vi "ContinueCompare_DetectEvent.vi"(3 "status":bool, 4 "error in (no error)":errorcluster, 5 "Task ID":u32) -> (0 "continue compare data":T1, 1 "error out":errorcluster, 2 "Task ID out":u32)   [LabVIEW 2015]
panel:
  in  "pattern match count":i32
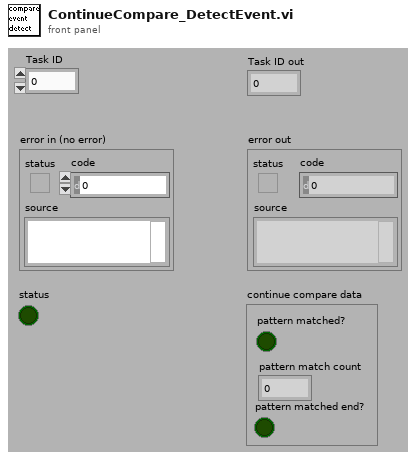
[diagram p1: front panel]
types:
  T1 = cluster{"pattern matched?":bool, "pattern matched end?":bool, "pattern match count":dbl}
  T2 = cluster{"pattern matched?":bool, "pattern matched end?":bool, "pattern match count":i32}
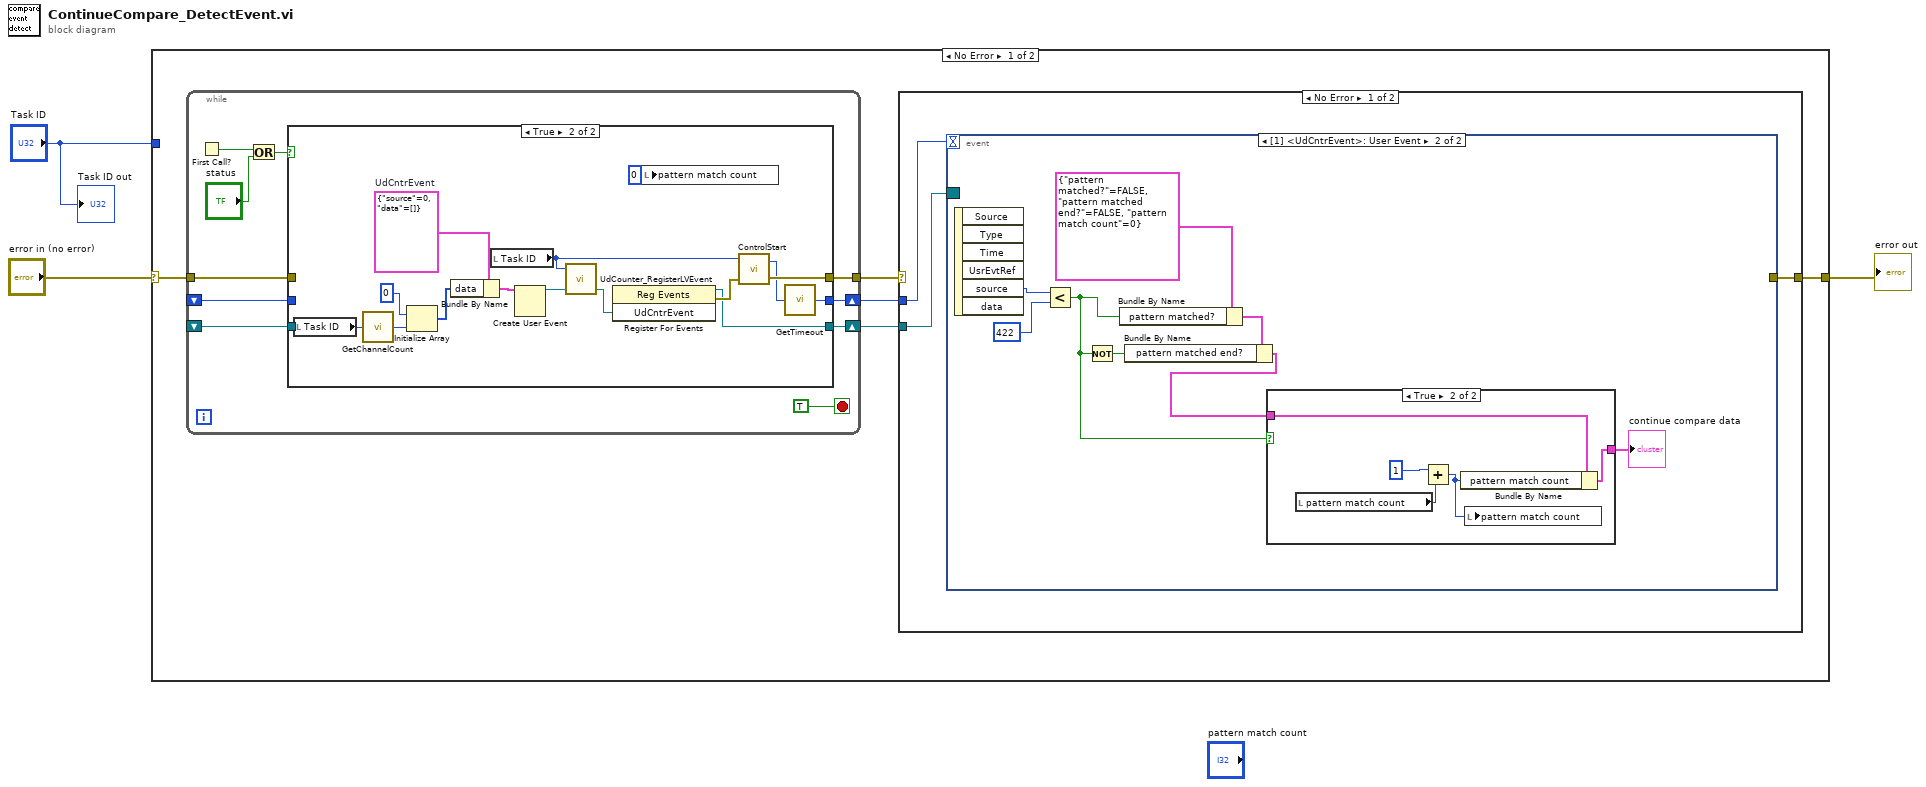
[diagram p0: block diagram]
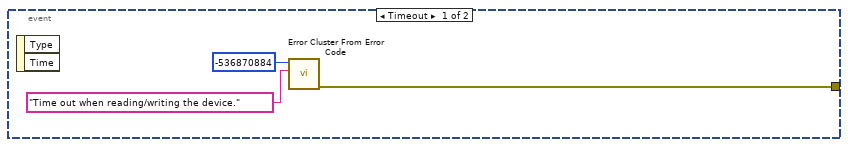
[diagram p2: hidden frame]
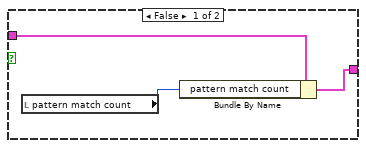
[diagram p3: hidden frame]
diagram:
  n1 = case shown="No Error" "error in (no error)" {
    selector: "error in (no error)" -> [w8 w60]
    tunnel: [w6 w60] -> w2
    tunnel: "Task ID" -> [_ _]
    frame No Error {
      n2 = while {
        tunnel: w8 -> [w37]
        tunnel: [w36] -> w7
        shift-right: [w34] -> w4
        shift-left: _ -> [w35]
        shift-right: [w32] -> w5
        shift-left: _ -> [w33]
        stop <- TRUE stop-if-true
        n3 = First Call?() -> (First Call?: T/F=w40:bool)
        n4 = Or(x=w40, y="status") -> (x .or. y?=w38:bool)
        n5 = case shown="True" w38 {
          tunnel: w37 -> [w44 _]
          tunnel: [w44 w52] -> w36
          tunnel: w35 -> [w43 _]
          tunnel: [w43 w51] -> w34
          tunnel: [w42 w50] -> w32
          tunnel: w33 -> [w42 _]
          frame False {
          }
          frame True {
            w56 = cluster{"source":i64, "data":i32[]} {"source"=0, "data"=[]}  # UdCntrEvent
            n6 = local read "Task ID"() -> (w59:u32)
            n7 = call "GetChannelCount.vi"("Task ID"=w59) -> ("return type"=w58:i32)
            n8 = Initialize Array(0 ("element"), w58) -> (w55:i32[])
            n9 = Bundle By Name(cluster=w56, "data"=w55) -> (w54:cluster{"source":i64, "data":i32[]})
            n10 = local read "Task ID"() -> (w48:u32)
            n11 = Create User Event(user event datatype=w54) -> (user event=w46:refnum<user-event>)  [unwired: 1 in, 1 out]
            n12 = call "UdCounter_RegisterLVEvent.vi"("UdCntrEvent"=w46, "Task ID"=w48) -> ("UdCntrEvent"=w45:refnum<user-event>)  [unwired: 1 in, 2 out]
            n13 = register-events(w45) -> (reference out=w51:refnum<event-registration>, error out=w53:errorcluster)  [unwired: 2 in]
            n14 = local write "pattern match count"(0 ("pattern match count")) -> ()
            n15 = call "ControlStart.vi"("error in (no error)"=w53, "Task ID"=w48) -> ("error out"=w52:errorcluster, "Task ID"=w49:u32)  [unwired: 1 out]
            n16 = call "GetTimeout.vi"("Task ID"=w49) -> ("return type"=w50:i32)
          }
        }
      }
      n17 = case shown="No Error" w7 {
        selector: w7 -> [_ w31]
        tunnel: [w9 w31] -> w6
        tunnel: w5 -> [w11 _]
        tunnel: w4 -> [w10 _]
        frame No Error {
          n18 = event shown="[1] <UdCntrEvent>: User Event" {
            selector: w10 -> [_ _]
            dyn-events: _ -> [_ _]
            timeout: w11 -> [_ _]
            tunnel: [w13 _] -> w9
            event Timeout {
              n19 = event-data() -> ()  [unwired: 3 out]
              n20 = call <vilib>:"Error Cluster From Error Code.vi"("error message (\"\")"="Time out when reading/writing the device." ("error message (\"\")"), "error code (0)"=-536870884) -> ("error out"=w13:errorcluster)  [unwired: 2 in, 5 out]
            }
            event User Event {
              n21 = event-data() -> ("source"=w21:i64)  [unwired: 6 out]
              n22 = Less?(x=w21, y=422) -> (x < y?=w17:bool)
              n23 = Not(x=w17) -> (.not. x?=w18:bool)
              n24 = Bundle By Name(cluster=T2 {"pattern matched?"=FALSE, "pattern matched end?"=FALSE, "pattern match count"=0}, "pattern matched?"=w17) -> (w19:T2)
              n25 = Bundle By Name(cluster=w19, "pattern matched end?"=w18) -> (w16:T2)
              n26 = case shown="True" w17 {
                tunnel: w16 -> [w25 w28]
                tunnel: [w24 w27] -> w15
                frame False {
                  n27 = local read "pattern match count"() -> (w23:i32)
                  n28 = Bundle By Name(cluster=w25, "pattern match count"=w23) -> (w24:T2)
                }
                frame True {
                  n29 = local read "pattern match count"() -> (w30:i32)
                  n30 = Add(x=1, y=w30) -> (x+y=w26:i32)
                  n31 = Bundle By Name(cluster=w28, "pattern match count"=w26) -> (w27:T2)
                  n32 = local write "pattern match count"(w26) -> ()
                }
              }
              "continue compare data" <- w15
            }
          }
        }
        frame Error {
        }
      }
    }
    frame Error {
    }
  }
  "error out" <- w2
  "Task ID out" <- "Task ID"
